vi "Get Position.vi"(8 "error in (no error)":errorcluster, 11 "Stage Controller in":refnum<class "Stage Controller.lvclass">) -> (0 "error out":errorcluster, 1 "Y (mm)":dbl, 2 "X (mm)":dbl, 3 "Stage Controller out":refnum<class "Stage Controller.lvclass">)   [LabVIEW 2018, in "Stage Controller.lvlib" / "Stage Controller.lvclass"]
uses:
  Stage Controller.lvclass
  Stage Controller.lvclass/Stage Controller.ctl
  <instrlib>/ASI TG-1000/Public/Utility/Axis Name.ctl
  <vilib>/Utility/error.llb/Error Cluster From Error Code.vi
  <vilib>/ErrorRing/Error Ring.xnode
  Microscope/ti2lv/ti2lv.lvlib
  <instrlib>/ASI TG-1000/ASI TG-1000.lvlib
  Stage Controller.lvlib
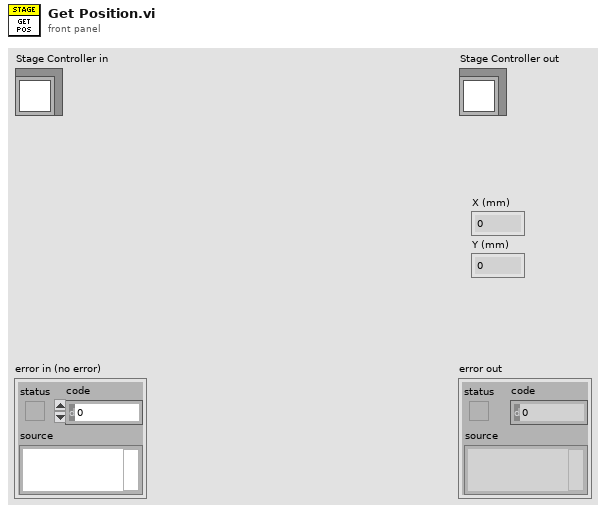
[diagram p1: front panel]
types:
  T1 = typedef "Stage Controller.lvlib/ASI TG-1000.lvlib/Axis Name.ctl" = enum8{"undefined", "A", "B", "C", "D", "E", "F", "G", "H", "I", "J", "K", "L", "M", "N", "O", "P", "Q", "R", "S", "T", "U", "V", "W", "X", "Y", "Z"}
  T2 = enum16{"Disabled", "ESP301", "Ti2", "Ludl", "ASI"}
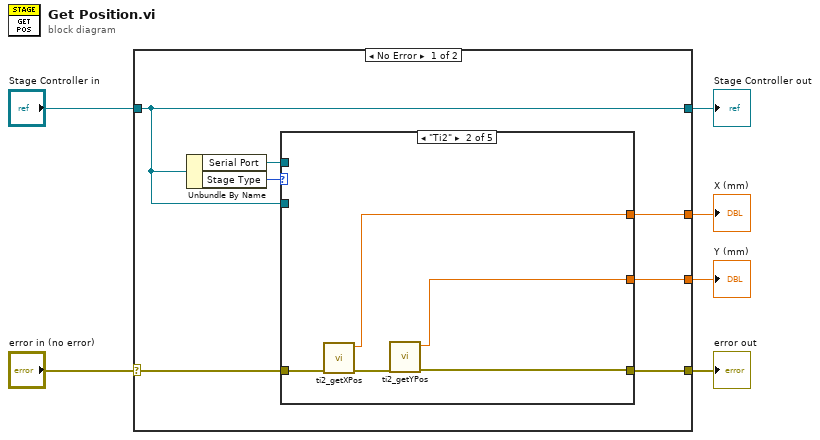
[diagram p0: block diagram]
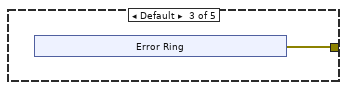
[diagram p3: hidden frame]
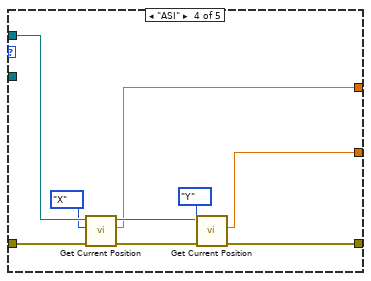
[diagram p4: hidden frame]
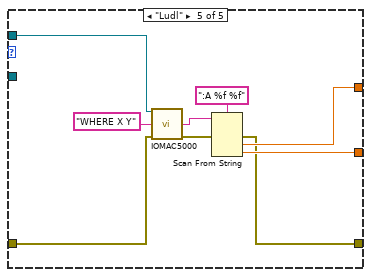
[diagram p5: hidden frame]
diagram:
  n1 = case shown="No Error" "error in (no error)" {
    selector: "error in (no error)" -> [w12 w44]
    tunnel: [w11 w44] -> w5
    tunnel: [w10 w43] -> w3
    tunnel: "Stage Controller in" -> [w10 w43]
    tunnel: [w8 _] -> w2
    tunnel: [w7 _] -> w1
    frame No Error {
      n2 = Unbundle By Name(w10) -> ("Serial Port"=w9:refnum<visa-resource-name>, "Stage Type"=w13:T2)
      n3 = case shown="\"Ti2\"" w13 {
        tunnel: w12 -> [w14 w19 _ w33 w41]
        tunnel: [w14 w17 w20 w31 w35] -> w11
        tunnel: w10 -> [_ _ _ _ _]
        tunnel: w9 -> [_ _ _ w30 w42]
        tunnel: [_ w16 _ w26 w38] -> w8
        tunnel: [_ w15 _ w25 w37] -> w7
        frame "Disabled" {
        }
        frame "Ti2" {
          n4 = call "ti2_getXPos.vi"("error in (no error)"=w19) -> ("error out"=w18:errorcluster, "x Position (um)"=w16:dbl)  [unwired: 9 in]
          n5 = call "ti2_getYPos.vi"("error in (no error)"=w18) -> ("error out"=w17:errorcluster, "y Position (um)"=w15:dbl)  [unwired: 9 in]
        }
        frame Default {
          n6 = xnode "Error Ring"() -> ("error out"=w20:errorcluster)
        }
        frame "ASI" {
          n7 = call <instrlib>:"Get Current Position.vi"("error in (no error)"=w33, "Axis"=Axis_Name."X", "VISA in"=w30) -> ("error out"=w32:errorcluster, "position [internal units]"=w26:dbl, "VISA out"=w27:refnum<visa-resource-name>)  [unwired: 6 in]
          n8 = call <instrlib>:"Get Current Position.vi"("error in (no error)"=w32, "Axis"=Axis_Name."Y", "VISA in"=w27) -> ("error out"=w31:errorcluster, "position [internal units]"=w25:dbl)  [unwired: 6 in, 1 out]
        }
        frame "Ludl" {
          n9 = call "IOMAC5000.vi"("VISA  IN"=w42, "Command (to ctlr)"="WHERE X Y" ("format string"), "error in"=w41) -> ("Raw Response"=w39:string, "error out"=w34:errorcluster)  [unwired: 9 in, 2 out]
          n10 = Scan From String(format string=":A %f %f", input string=w39, error in=w34) -> (error out=w35:errorcluster, output 1=w38:dbl, output 2=w37:dbl)  [unwired: 3 in, 2 out]
        }
      }
    }
    frame Error {
    }
  }
  "error out" <- w5
  "Stage Controller out" <- w3
  "X (mm)" <- w2
  "Y (mm)" <- w1
